vi "Configure Under Voltage Type.vi"(6 "Settle (1mS)":u32=1, 7 "Under Voltage Type  (0: UVL)":u16(ring) items=["UVL", "UVP"], 8 "error in (no error)":errorcluster, 10 "UV Level (0V)":dbl format="%.4f", 11 "VISA resource name":refnum<visa-resource-name>) -> (0 "error out":errorcluster, 3 "VISA resource name out":refnum<visa-resource-name>)   [LabVIEW 2013, in "TDK-Lambda Z.lvlib"]
doc: "Sets the under voltage protection (UVP) status of the power supply. If the UVP status is UVP, then the under voltage protection is enabled. If the UVP status is UVL, then the under voltage protection is disabled and only under voltage level (UVL) is enabled\n\nNote: This VI will wait for \"Settle\" milliseconds after setting the limit to allow the output to reach the new setting. If unwired, there will be no delay"
uses:
  TDK-Lambda Z.lvlib
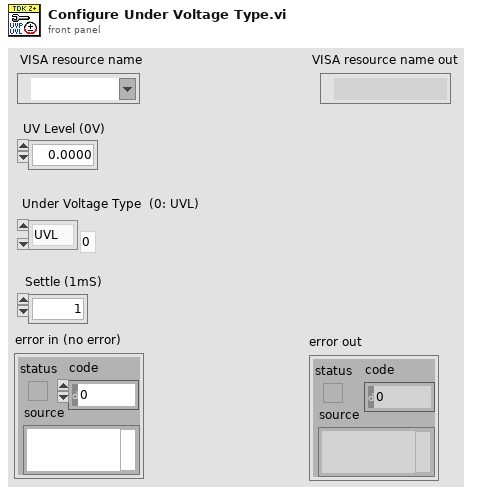
[diagram p1: front panel]
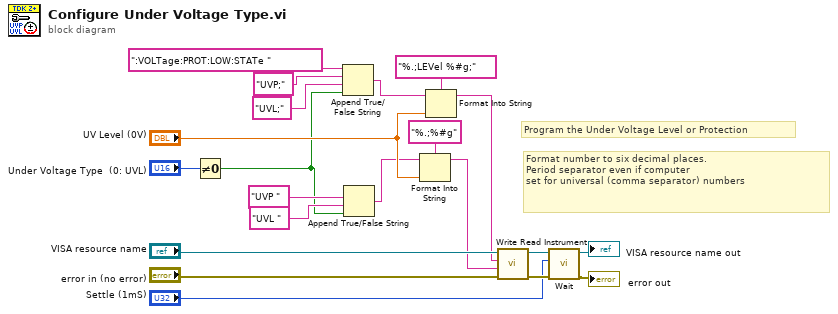
[diagram p0: block diagram]
diagram:
  # "Format number to six decimal places.\nPeriod separator even if computer \nset for universal (comma separator) numbers"
  # "Program the Under Voltage Level or Protection"
  n1 = Not Equal To 0?(x="Under Voltage Type  (0: UVL)") -> (x != 0?=w1:bool)
  n2 = Append True/False String(1:w1, 2:"UVL;" ("true string"), 3:"UVP;" ("true string"), 4:":VOLTage:PROT:LOW:STATe " ("format string")) -> (0:w7:string)
  n3 = Append True/False String(1:w1, 2:"UVL " ("true string"), 3:"UVP " ("true string")) -> (0:w4:string)  [unwired: 1 in]
  n4 = Format Into String(format string="%.;%#g", initial string=w4, "UV Level (0V)") -> (resulting string=w17:string)  [unwired: 1 in, 1 out]
  n5 = Format Into String(format string="%.;LEVel %#g;", initial string=w7, "UV Level (0V)") -> (resulting string=w19:string)  [unwired: 1 in, 1 out]
  n6 = call "Write Read Instrument.vi"("error in (no error)"="error in (no error)", "GEN  Write Command/Query"=w17, "SCPI  Write Command/Query"=w19, "VISA resource name"="VISA resource name") -> ("error out"=w14:errorcluster, "VISA resource name out"=w15:refnum<visa-resource-name>)  [unwired: 5 in, 1 out]
  n7 = call "Wait.vi"("error in (no error)"=w14, "Wait (1mS)"="Settle (1mS)", "VISA resource name"=w15) -> ("error out"=→"error out":errorcluster, "VISA resource name out"=→"VISA resource name out":refnum<visa-resource-name>)  [unwired: 7 in]
